vi "PGS.vi"(0 "System no.":i32=1 min=1 max=4 step=1, 2 "Nexline channel":string[](array[string]), 3 "All channels?":bool, 4 "Channel identifier?":bool=TRUE, 5 "error in":errorcluster) -> (19 "error out":errorcluster)   [LabVIEW 2026]
doc: "Makes the current settings of the parameters for the Nexline channel piezo gain correction (APG) default by writing them to the EPROM.\n\nE-755: If All channels? = TRUE, then Channel identifier? must be FALSE. Command is available in command level 1 only (see CCL.vi). Command not available for E-755.101."
panel:
  # "Makes the current settings of the parameters for \nthe Nexline channel piezo gain correction (APG) \ndefault by writing them to the EPROM."
  # "If all channels: use"
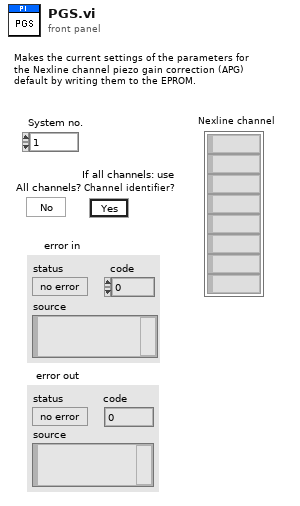
[diagram p1: front panel]
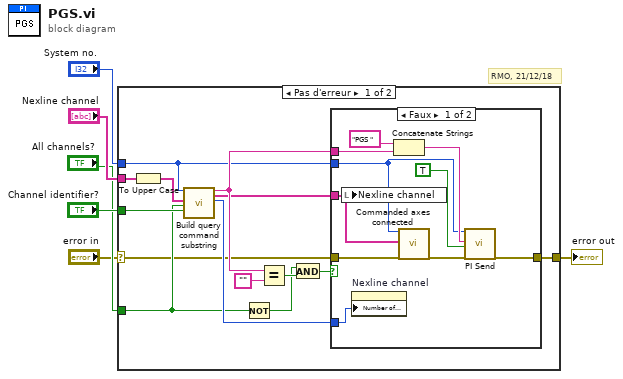
[diagram p0: block diagram]
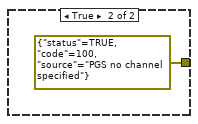
[diagram p2: hidden frame]
diagram:
  # "RMO, 21/12/18"
  n1 = case shown="Pas d'erreur" "error in" {
    selector: "error in" -> [w7 w32]
    tunnel: "Nexline channel" -> [w20 _]
    tunnel: "Channel identifier?" -> [w17 _]
    tunnel: "System no." -> [w15 _]
    tunnel: "All channels?" -> [w11 _]
    tunnel: [w9 w32] -> w2
    frame No Error {
      n2 = To Upper Case(1:w20) -> (0:w18:string[])
      n3 = call "Build query command substring.vi"("System no."=w15, "Axes to query in"=w18, "Query\nAll axes?"=w11, "For all axes: use\nAxis identifier?"=w17) -> ("Command substring"=w16:string, "Axes to query out"=w14:string[], "Number of rows"=w13:u32)  [unwired: 2 in, 11 out]
      n4 = Not(x=w11) -> (.not. x?=w10:bool)
      n5 = Equal?(x=w16, y="" ("x")) -> (x = y?=w12:bool)
      n6 = And(x=w10, y=w12) -> (x .and. y?=w8:bool)
      n7 = case shown="Faux" w8 {
        tunnel: w7 -> [w27 _]
        tunnel: w16 -> [w26 _]
        tunnel: w15 -> [w25 _]
        tunnel: w14 -> [w24 _]
        tunnel: w13 -> [w22 _]
        tunnel: [w21 errorcluster {"status"=TRUE, "code"=100, "source"="PGS no channel specified"} ("error out")] -> w9
        frame False {
          n8 = local write "Nexline channel"(w24) -> ()
          n9 = property on="Nexline channel" class="Tabl (strict)"("Number of Rows"=w22) -> ()  [unwired: 2 in, 2 out]
          n10 = Concatenate Strings("PGS ", w26) -> (w28:string)
          n11 = call "Commanded axes connected.vi"("System no."=w25, "Commanded axes"=w24, "error in"=w27) -> ("error out"=w23:errorcluster)  [unwired: 1 in, 15 out]
          n12 = call "PI Send.vi"("System no."=w25, "String to send"=w28, "Attach termination char.?"=TRUE ("Attach Linefeed?"), "error in"=w23) -> ("error out"=w21:errorcluster)  [unwired: 2 in, 13 out]
        }
        frame True {
        }
      }
    }
    frame Error {
    }
  }
  "error out" <- w2
